vi "File_to_Logcluster.vi"(0 "Cyphered text":string, 11 "error in (no error)":errorcluster) -> (4 "Log Cluster Out":T1, 15 "error out":errorcluster)   [LabVIEW 2012]
uses:
  typedef/Log_User_Data.ctl
  typedef/User Accounts.ctl
panel:
  in  "Log Cluster":T1
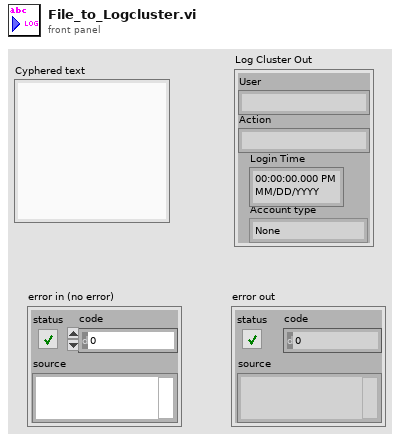
[diagram p1: front panel]
types:
  T1 = typedef "Log_User_Data.ctl" = cluster{"User":string, "Action":string, "Account type":T2, "Login Time ":timestamp}
  T2 = typedef "User Accounts.ctl" = enum16{"None", "User", "Admin"}
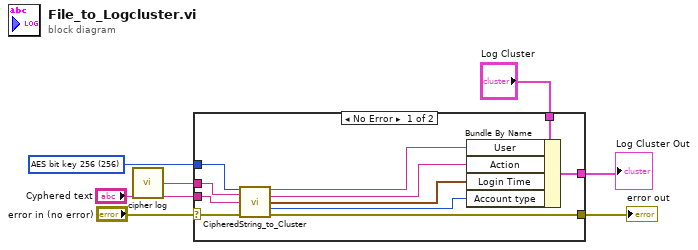
[diagram p0: block diagram]
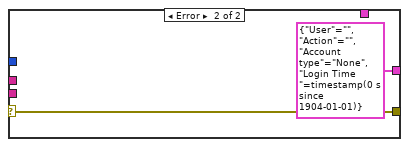
[diagram p2: hidden frame]
diagram:
  w5 = u16 256 items=["AES bit key 128"=128, "AES bit key 192"=192, "AES bit key 256"=256] ("BitKeyType (256)")
  n1 = call "cipher log.vi"() -> ("password to cipher log"=w2:string)  [unwired: 15 in]
  n2 = case shown="No Error" "error in (no error)" {
    selector: "error in (no error)" -> [w17 w20]
    tunnel: "Cyphered text" -> [w18 _]
    tunnel: [w9 w20] -> w6
    tunnel: w2 -> [w10 _]
    tunnel: w5 -> [w11 _]
    tunnel: "Log Cluster" -> [w16 _]
    tunnel: [w12 T1 {"User"="", "Action"="", "Account type"=enum."None", "Login Time "=timestamp(0 s since 1904-01-01)} ("Log Cluster")] -> w1
    frame No Error {
      n3 = call "CipheredString_to_Cluster.vi"("BitKeyType (256)"=w11, "password to cipher users"=w10, "Cyphered text"=w18, "error in (no error)"=w17) -> ("String 1"=w15:string, "String 2"=w8:string, "Time Stamp"=w13:timestamp, "Account"=w14:T2, "error out"=w9:errorcluster)  [unwired: 7 in]
      n4 = Bundle By Name(cluster=w16, "User"=w15, "Action"=w8, "Login Time"=w13, "Account type"=w14) -> (w12:T1)
    }
    frame Error {
    }
  }
  "error out" <- w6
  "Log Cluster Out" <- w1
